vi "Untitled_.vi"() -> ()   [LabVIEW 2010]
uses:
  <instrlib>/niScope/Controls/niScope vertical coupling.ctl
  <instrlib>/niScope/Controls/niScope trigger coupling.ctl
  <instrlib>/niScope/Controls/niScope trigger slope.ctl
  <instrlib>/niScope/Controls/niScope trigger source.ctl
  <instrlib>/niSync/niSync.llb/niSync Initialize (String).vi
  <instrlib>/niScope/Configure/Trigger/niScope Configure Trigger Edge.vi
  <instrlib>/niScope/Acquire/niScope Multi Read WDT.vi
panel:
  in  "Time Stamp":timestamp=timestamp(3347805600 s since 1904-01-01)
  out "x-y":dbl
  out "element":T1
  out "t0":timestamp
  out "error out":errorcluster
  out "time GPS":timestamp caption="time"
  out "Waveform Graph":waveform(dbl)[](graph)
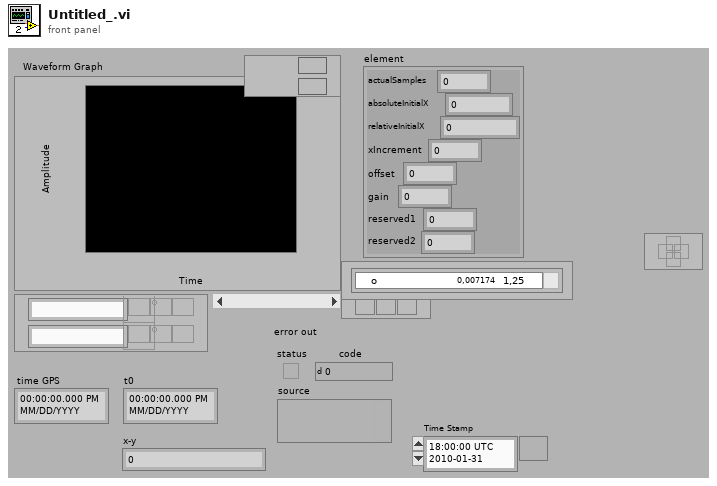
[diagram p1: front panel]
types:
  T1 = cluster{"actualSamples":i32, "absoluteInitialX":dbl, "relativeInitialX":dbl, "xIncrement":dbl, "offset":dbl, "gain":dbl, "reserved1":dbl, "reserved2":dbl}
  T2 = typedef "niScope trigger source.ctl" = string
  T3 = typedef "niScope trigger slope.ctl" = i32
  T4 = typedef "niScope trigger coupling.ctl" = u16
  T5 = typedef "niScope vertical coupling.ctl" = i32
  T6 = cluster{"actualSamples":i32, "absoluteInitialX":dbl, "relativeInitialX":dbl, "xIncrement":dbl, "offset":dbl, "gain":dbl, "reserved1":dbl, "reserved2":dbl}[]
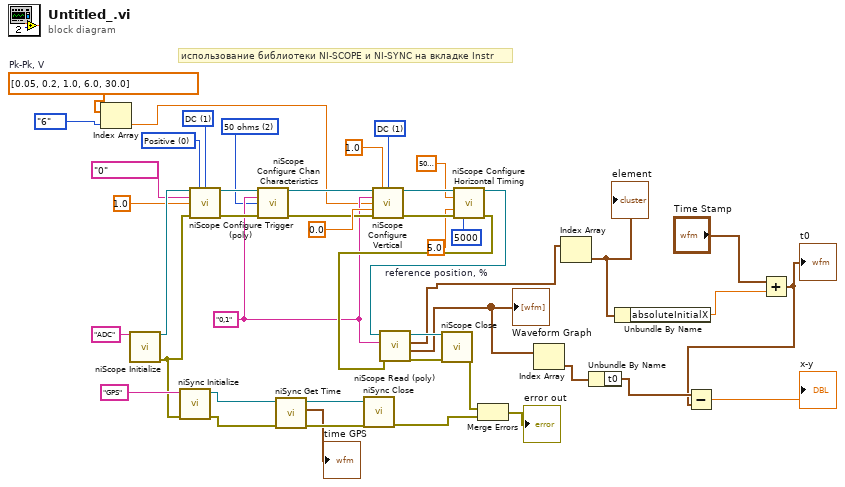
[diagram p0: block diagram]
diagram:
  w3 = dbl[] [0.05, 0.2, 1.0, 6.0, 30.0]  # Pk-Pk, V
  w16 = T3 0 items=["Positive", "Negative"] ("trigger slope")
  w17 = T4 1 items=["AC"=0, "DC"=1, "HF Reject"=3, "LF Reject"=4, "AC Plus HF Reject"=1001] ("trigger coupling")
  w18 = u32 2 items=["1 mega ohm"=0, "50 ohms"=2] ("input impedance")
  w26 = 5.0  # reference position, %
  w31 = T5 1 items=["AC", "DC", "Ground"] ("vertical coupling")
  w19 = "0,1" ("channels")
  # "использование библиотеки NI-SCOPE и NI-SYNC на вкладке Instr"
  n1 = Index Array(array=w3, index=enum16{"1/20", "1/5", "1", "6", "30"}."6") -> (element=w1:dbl)
  n2 = call <instrlib>:"niScope Initialize.vi"("resource name"="ADC") -> ("instrument handle"=w32:refnum<k15>, "error out"=w24:errorcluster)  [unwired: 13 in]
  n3 = call-poly <instrlib>:"niSync Initialize.vi"("error in (no error)"=w24, "resource name"="GPS") -> ("error out"=w41:errorcluster, "instrument handle out"=w42:refnum<k15>)  [unwired: 8 in]
  n4 = call-poly <instrlib>:"niScope Configure Trigger (poly).vi"("instrument handle"=w32, "trigger slope"=w16, "trigger coupling"=w17, "trigger source"=T2 "0", "trigger level"=1.0, "error in"=w24) -> ("instrument handle out"=w23:refnum<k15>, "error out"=w22:errorcluster)  [unwired: 8 in]
  n5 = call <instrlib>:"niScope Configure Chan Characteristics.vi"("instrument handle"=w23, "channels"=w19, "input impedance"=w18, "error in"=w22) -> ("instrument handle out"=w20:refnum<k15>, "error out"=w21:errorcluster)  [unwired: 10 in]
  n6 = call <instrlib>:"niSync Get Time.vi"("error in (no error)"=w41, "instrument handle"=w42) -> ("error out"=w39:errorcluster, "time"=→"time GPS":timestamp, "instrument handle out"=w40:refnum<k15>)  [unwired: 5 in]
  n7 = call <instrlib>:"niSync Close.vi"("error in (no error)"=w39, "instrument handle"=w40) -> ("error out"=w36:errorcluster)  [unwired: 9 in]
  n8 = call <instrlib>:"niScope Configure Vertical.vi"("instrument handle"=w20, "probe attenuation"=1.0, "vertical coupling"=w31, "channels"=w19, "vertical range"=w1, "vertical offset"=0.0, "error in"=w21) -> ("instrument handle out"=w33:refnum<k15>, "error out"=w34:errorcluster)  [unwired: 7 in]
  n9 = call <instrlib>:"niScope Configure Horizontal Timing.vi"("instrument handle"=w33, "min sample rate"=5000000.0, "reference position"=w26, "error in"=w34, "min record length"=5000) -> ("instrument handle out"=w27:refnum<k15>, "error out"=w28:errorcluster)  [unwired: 9 in]
  n10 = call-poly <instrlib>:"niScope Read (poly).vi"("error in"=w28, "channels"=w19, "instrument handle"=w27) -> ("error out"=w43:errorcluster, "wfm"=w10:waveform(dbl)[], "wfm info"=w12:T6, "instrument handle out"=w44:refnum<k15>)  [unwired: 5 in]
  "Waveform Graph" <- w10
  n11 = call <instrlib>:"niScope Close.vi"("instrument handle"=w44, "error in"=w43) -> ("error out"=w37:errorcluster)  [unwired: 13 in]
  n12 = Merge Errors(w37, w36) -> (→"error out":errorcluster)
  n13 = Index Array(array=w10) -> (element=w9:waveform(dbl))  [unwired: 1 in]
  n14 = Index Array(array=w12) -> (element=w11:T1)  [unwired: 1 in]
  "element" <- w11
  n15 = Unbundle By Name(w9) -> ("t0"=w8:timestamp)
  n16 = Unbundle By Name(w11) -> ("absoluteInitialX"=w5:dbl)
  n17 = Add(x="Time Stamp", y=w5) -> (x+y=w4:timestamp)
  "t0" <- w4
  n18 = Subtract(x=w8, y=w4) -> (x-y=→"x-y":dbl)
